vi "Set Server Address.vi"(10 "Server Address":string, 11 "OOP Server in":refnum<class "OCV.lvclass">) -> (3 "OOP Server out":refnum<class "OCV.lvclass">)   [LabVIEW 2019, in "OCV.lvlib" / "OCV.lvclass"]
uses:
  OCV.lvclass
  OCV.lvclass/OCV.ctl
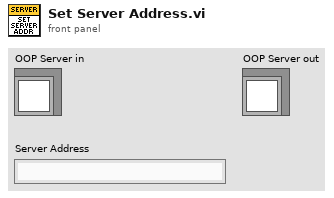
[diagram p1: front panel]
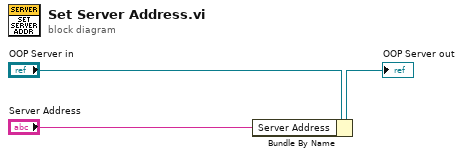
[diagram p0: block diagram]
diagram:
  n1 = Bundle By Name(cluster="OOP Server in", "Server Address"="Server Address") -> (→"OOP Server out":refnum<class "OCV.lvclass">)
